vi "Tool selector (SubVI).vi"(3 "Z, Hight":dbl format="%#_13g", 4 "Obejct length":dbl, 5 "Assignment -Task - Tool":string) -> (0 "Tool 2":string, 1 "Tool":dbl, 2 "Assignment - Task":string)   [LabVIEW 2022 SP3]
doc: "Selecting tool from object length.\nCorrecting height from user input."
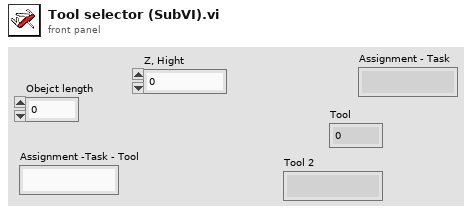
[diagram p1: front panel]
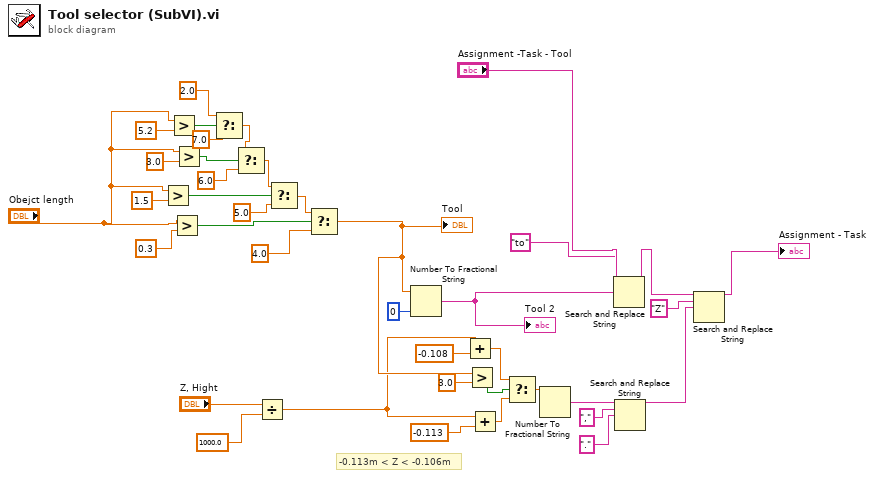
[diagram p0: block diagram]
diagram:
  # "-0.113m < Z < -0.106m"
  n1 = Greater?(x="Obejct length", y=1.5) -> (0:w32:bool)
  n2 = Greater?(x="Obejct length", y=5.2) -> (0:w29:bool)
  n3 = Greater?(x="Obejct length", y=0.3 ("upper limit")) -> (0:w30:bool)
  n4 = Greater?(x="Obejct length", y=3.0) -> (0:w34:bool)
  n5 = Select(t=2.0, s=w29, f=7.0) -> (s? t:f=w38:dbl)
  n6 = Select(t=w38, s=w34, f=6.0) -> (s? t:f=w35:dbl)
  n7 = Divide(x="Z, Hight", y=1000.0) -> (x/y=w14:dbl)
  n8 = Select(t=w35, s=w32, f=5.0) -> (s? t:f=w33:dbl)
  n9 = Select(t=w33, s=w30, f=4.0) -> (s? t:f=w16:dbl)
  "Tool" <- w16
  n10 = Number To Fractional String(number=w16, precision (6)=i16 0) -> (F-format string=w28:string)  [unwired: 2 in]
  "Tool 2" <- w28
  n11 = Add(x=w14, y=-0.108) -> (x+y=w11:dbl)
  n12 = Greater?(x=w16, y=3.0) -> (0:w9:bool)
  n13 = Add(x=w14, y=-0.113 ("Z, Hight")) -> (x+y=w10:dbl)
  n14 = Select(t=w11, s=w9, f=w10) -> (s? t:f=w12:dbl)
  n15 = Number To Fractional String(number=w12) -> (F-format string=w19:string)  [unwired: 3 in]
  n16 = Search and Replace String(input string="Assignment -Task - Tool", search string="to", replace string=w28) -> (result string=w18:string)  [unwired: 5 in, 3 out]
  n17 = Search and Replace String(input string=w19, search string=",", replace string="." ("replace string (\"\")")) -> (result string=w8:string)  [unwired: 5 in, 3 out]
  n18 = Search and Replace String(input string=w18, search string="Z", replace string=w8) -> (result string=→"Assignment - Task":string)  [unwired: 5 in, 3 out]
